vi "Initialise.vi"(8 "error in (no error)":errorcluster, 10 "Message in":refnum<class "InitialiseMessage.lvclass">, 11 "Retiga in":refnum<class "Retiga.lvclass">) -> (0 "error out":errorcluster, 3 "Retiga out":refnum<class "Retiga.lvclass">)   [LabVIEW 2012, in "Retiga.lvclass"]
doc: "This method is called when an initialise message is received. It mainly initialises the RabbitMQ connectivity. \n\nOverride this method when your component needs special initialisation (e.g. of software or hardware resources). In that case, don't forget to call the parent for proper implementation. If your component owns subcomponents, they count as resources, so you have to initialise them by calling their own initialise functions"
uses:
  Retiga.lvclass
  <vilib>/Distrio/Murmex/InitialiseMessage/InitialiseMessage.lvclass
  <vilib>/Distrio/Murmex/Murmex/Murmex.lvclass
  Retiga.lvclass/Retiga.ctl
panel:
  # "This method is called when the INTIALISE\ntrigger is sent. \n\nOverride this method when your component needs to\nrespond to this trigger. \n\nCall parent for proper implementation"
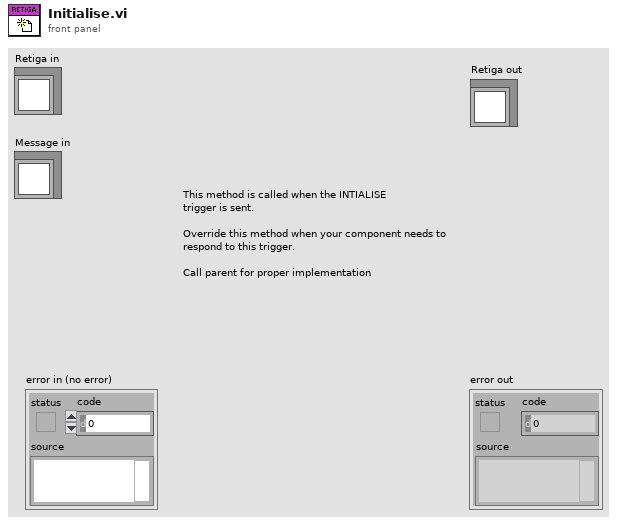
[diagram p1: front panel]
types:
  T1 = enum32{"gain", "offset", "exposure", "binning", "horizontal binning", "vertical binning", "readout speed", "trigger type", "lcd filter", "cooler", "exposure red", "exposure blue", "image format", "roi x", "roi y", "roi width", "roi height", "reserved1", "shutter state", "reserved2", "sync-b out", "reserved3", "intensifier gain", "trigger delay", "camera mode", "normalized gain", "normalized intenifier gain DB", "doPostProcessing", "postProcessGainRed", "postProcessGainGreen", "postProcessGainBlue", "postProcessBayerAlgorithm", "postProcessImageFormat", "fan", "blackout mode", "high sensitivity", "Readout Port", "EM Gain", "open delay", "close delay", "clearing mode"}
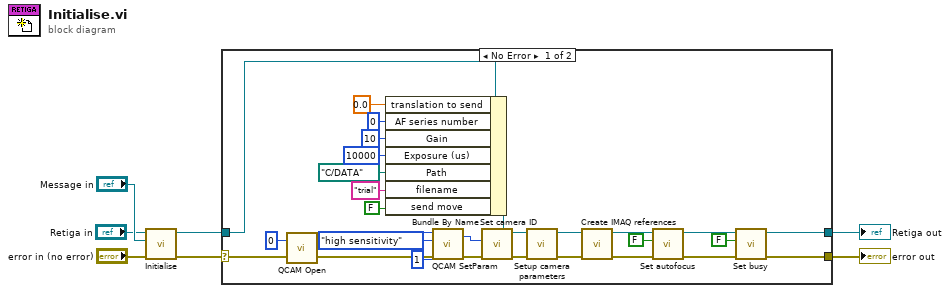
[diagram p0: block diagram]
diagram:
  n1 = call-parent "Initialise.vi"("error in (no error)"="error in (no error)", "Message in"="Message in", "Murmex in"="Retiga in") -> ("error out"=w4:errorcluster, "Murmex out"=w2:refnum<class "Retiga.lvclass">)  [unwired: 7 in]
  n2 = case shown="No Error" w4 {
    selector: w4 -> [w35 w38]
    tunnel: [w17 w38] -> w3
    tunnel: w2 -> [w34 w37]
    tunnel: [w19 w37] -> w1
    frame No Error {
      n3 = call <userlib>:"QCAM Open.vi"("error in (no error)"=w35, "cameraId"=u32 0) -> ("error out"=w12:errorcluster, "cameraId out"=w15:u32)
      n4 = Bundle By Name(cluster=w34, "translation to send"=dbl[unit] 0.0 ("runtime.translation to send"), "AF series number"=0 ("runtime.AF series number"), "Gain"=10 ("settings.Gain"), "Exposure (us)"=10000 ("settings.Exposure (us)"), "Path"=path "C:/DATA" ("settings.Path"), "filename"="trial" ("settings.filename"), "send move"=FALSE ("runtime.cross correlation.send move")) -> (w22:refnum<class "Retiga.lvclass">)
      n5 = call <userlib>:"QCAM SetParam.vi"("error in (no error)"=w12, "value"=1, "parameter key"=T1."high sensitivity", "cameraId"=w15) -> ("error out"=w13:errorcluster, "cameraId out"=w14:u32)
      n6 = call-dynamic "Set camera ID.vi"("error in (no error)"=w13, "camera ID"=w14, "Retiga in"=w22) -> ("error out"=w24:errorcluster, "Retiga out"=w23:refnum<class "Retiga.lvclass">)  [unwired: 7 in]
      n7 = call-dynamic "Setup camera parameters.vi"("error in (no error)"=w24, "Retiga in"=w23) -> ("error out"=w33:errorcluster, "Retiga out"=w32:refnum<class "Retiga.lvclass">)  [unwired: 8 in]
      n8 = call-dynamic "Create IMAQ references.vi"("error in (no error)"=w33, "Retiga in"=w32) -> ("error out"=w31:errorcluster, "Retiga out"=w30:refnum<class "Retiga.lvclass">)  [unwired: 8 in]
      n9 = call-dynamic "Set autofocus.vi"("error in (no error)"=w31, "autofocusing?"=FALSE, "Retiga in"=w30) -> ("error out"=w18:errorcluster, "Retiga out"=w20:refnum<class "Retiga.lvclass">)  [unwired: 7 in]
      n10 = call-dynamic "Set busy.vi"("error in (no error)"=w18, "busy?"=FALSE, "Retiga in"=w20) -> ("error out"=w17:errorcluster, "Retiga out"=w19:refnum<class "Retiga.lvclass">)  [unwired: 7 in]
    }
    frame Error {
    }
  }
  "error out" <- w3
  "Retiga out" <- w1
